vi "Production Mode Alt Gas.vi"() -> ()   [LabVIEW 2019]
uses:
  <vilib>/Instr/_visa.llb/VISA Configure Serial Port (Instr).vi
  <vilib>/regexp/Match Regular Expression.xnode
panel:
  in  "Gas Type":bool
  in  "Name":string
  in  "sMDT Code":string
  out "Previous\nTest Passed":bool
  out "Status":string
  in  "Start":bool
  out "Leak":string
  out "Pressure (mTorr)":dbl
  # "100% He"
  # "5% He"
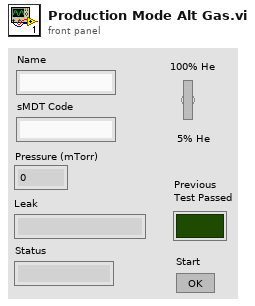
[diagram p1: front panel]
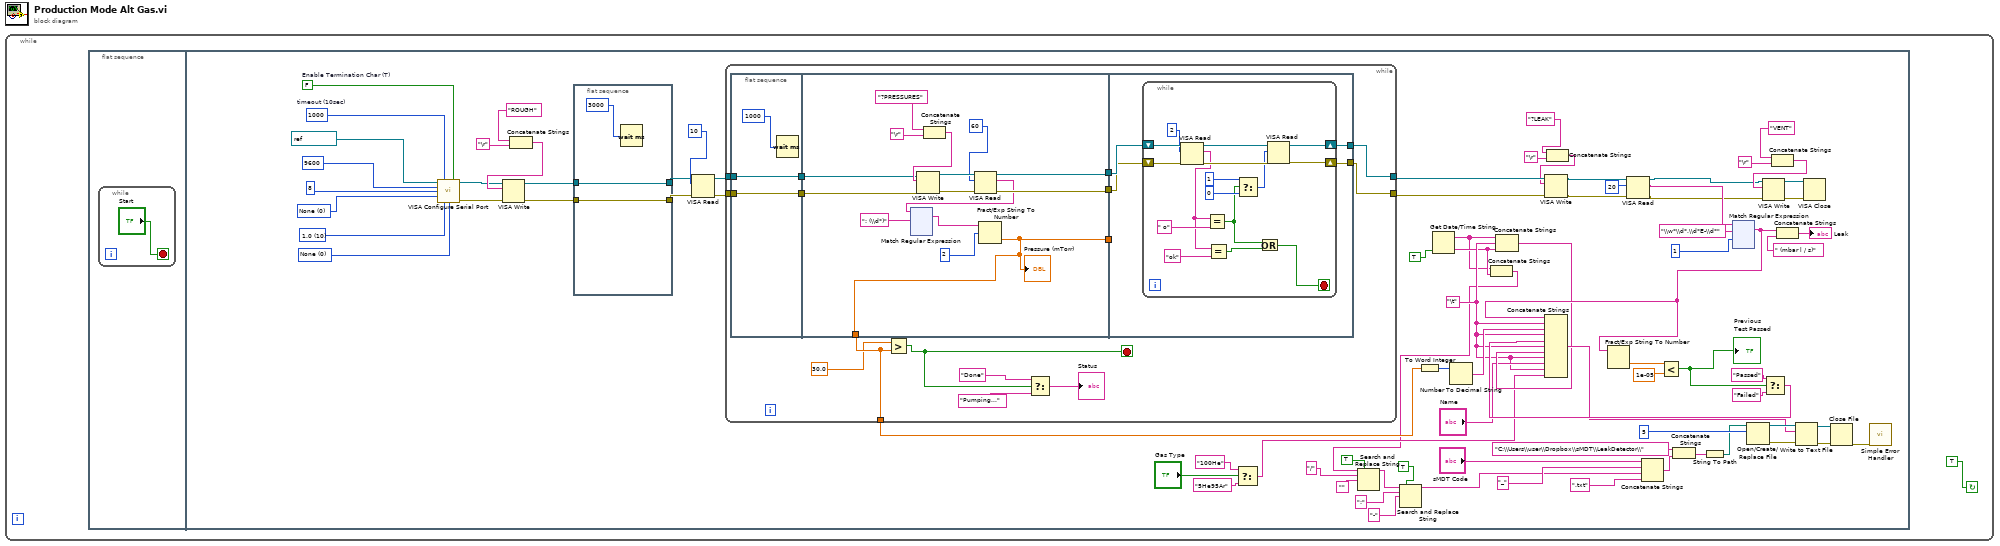
[diagram p0: block diagram]
diagram:
  n1 = while {
    stop <- TRUE continue-if-true
    n2 = flat-sequence {
      frame #0 {
        n3 = while {
          stop <- "Start" stop-if-true
        }
      }
      frame #1 {
        w16 = "\t"
        w79 = u16 0 items=["None"=0, "XON/XOFF"=1, "RTS/CTS"=2, "DTR/DSR"=4] ("flow control")
        w80 = u16 10 items=["1.0"=10, "1.5"=15, "2.0"=20] ("stop bits")
        w81 = u16 0 items=["None", "Odd", "Even", "Mark", "Space"] ("parity")
        w84 = FALSE  # Enable Termination Char (T)
        w85 = u32 1000  # timeout (10sec)
        n4 = call-poly "VISA Configure Serial Port"("VISA resource name"=refnum<visa-resource-name> "COM3", "timeout (10sec)"=w85, "Enable Termination\nChar (T)"=w84, "baud rate (9600)"=u32 9600 ("baud rate"), "data bits (8)"=u16 8 ("data bits"), "parity (0:none)"=w81, "stop bits (10: 1 bit)"=w80, "flow control (0:none)"=w79) -> ("VISA resource name out"=w18:refnum<visa-resource-name>, "error out"=w17:errorcluster)  [unwired: 6 in]
        n5 = Concatenate Strings("ROUGH", "\r") -> (w76:string)
        n6 = VISA Write(VISA resource name=w18, write buffer=w76, error in (no error)=w17) -> (VISA resource name out=w70:refnum<visa-resource-name>, error out=w69:errorcluster)  [unwired: 1 out]
        n7 = flat-sequence {
          tunnel: w70 -> [w367]
          tunnel: w69 -> [w368]
          tunnel: [w368] -> w66
          tunnel: [w367] -> w67
          frame #0 {
            n8 = Wait (ms)(milliseconds to wait=3000) -> ()  [unwired: 1 out]
          }
        }
        n9 = VISA Read(VISA resource name=w67, byte count=10, error in (no error)=w66) -> (VISA resource name out=w64:refnum<visa-resource-name>, error out=w65:errorcluster)  [unwired: 2 out]
        n10 = while {
          tunnel: w64 -> [w100]
          tunnel: w65 -> [w99]
          tunnel: [w88] -> w55
          tunnel: [w87] -> w54
          tunnel: [w92] -> w31
          stop <- w93 stop-if-true
          n11 = flat-sequence {
            tunnel: w100 -> [w103]
            tunnel: w99 -> [w102]
            tunnel: [w103] -> w98
            tunnel: [w102] -> w97
            tunnel: w98 -> [w112]
            tunnel: w97 -> [w111]
            tunnel: [w105] -> w92
            tunnel: [w109] -> w91
            tunnel: [w110] -> w90
            tunnel: [w105] -> w89
            tunnel: w91 -> [w235]
            tunnel: w90 -> [w236]
            tunnel: w89 -> [_]
            tunnel: [w234] -> w88
            tunnel: [w233] -> w87
            frame #0 {
              n12 = Wait (ms)(milliseconds to wait=1000) -> ()  [unwired: 1 out]
            }
            frame #1 {
              n13 = Concatenate Strings("?PRESSURES", "\r") -> (w113:string)
              n14 = VISA Write(VISA resource name=w112, write buffer=w113, error in (no error)=w111) -> (VISA resource name out=w118:refnum<visa-resource-name>, error out=w117:errorcluster)  [unwired: 1 out]
              n15 = VISA Read(VISA resource name=w118, byte count=60, error in (no error)=w117) -> (VISA resource name out=w110:refnum<visa-resource-name>, read buffer=w104:string, error out=w109:errorcluster)  [unwired: 1 out]
              n16 = xnode "Match Regular Expression"("input string"=w104, "regular expression"=": (\\d*)") -> ("whole match"=w108:string)  [unwired: 4 in, 4 out]
              n17 = Fract/Exp String To Number(string=w108, offset=2) -> (number=w105:dbl)  [unwired: 2 in, 1 out]
              "Pressure (mTorr)" <- w105
            }
            frame #2 {
              n18 = while {
                shift-right: [w246] -> w234
                shift-left: w236 -> [w252]
                shift-right: [w247] -> w233
                shift-left: w235 -> [w249]
                stop <- w237 stop-if-true
                n19 = VISA Read(VISA resource name=w252, byte count=2, error in (no error)=w249) -> (VISA resource name out=w250:refnum<visa-resource-name>, read buffer=w240:string, error out=w248:errorcluster)  [unwired: 1 out]
                n20 = Equal?(x=w240, y=" o") -> (x = y?=w238:bool)
                n21 = Equal?(x=w240, y="ok") -> (x = y?=w239:bool)
                n22 = Select(t=1, s=w238, f=0) -> (s? t:f=w243:i32)
                n23 = Or(x=w238, y=w239) -> (x .or. y?=w237:bool)
                n24 = VISA Read(VISA resource name=w250, byte count=w243, error in (no error)=w248) -> (VISA resource name out=w246:refnum<visa-resource-name>, error out=w247:errorcluster)  [unwired: 2 out]
              }
            }
          }
          n25 = Greater?(x=30.0 ("Pump Pressure"), y=w92) -> (0:w93:bool)
          n26 = Select(t="Done", s=w93, f="Pumping...") -> (s? t:f=→"Status":string)
        }
        n27 = Select(t="100He", s="Gas Type", f="5He95Ar") -> (s? t:f=w12:string)
        n28 = To Word Integer(number=w31) -> (16bit integer=w30:i16)
        n29 = Get Date/Time String(want seconds? (F)=TRUE) -> (date string=w9:string, time string=w10:string)  [unwired: 2 in]
        n30 = Number To Decimal String(number=w30) -> (decimal integer string=w27:string)  [unwired: 1 in]
        n31 = Concatenate Strings(w9, w10) -> (w8:string)
        n32 = Search and Replace String(replace all?=TRUE, input string=w8, search string="/", replace string="") -> (result string=w3:string)  [unwired: 4 in, 3 out]
        n33 = Search and Replace String(replace all?=TRUE, input string=w3, search string=":", replace string="-") -> (result string=w7:string)  [unwired: 4 in, 3 out]
        n34 = Concatenate Strings(w9, w16, w10) -> (w24:string)
        n35 = Concatenate Strings("?LEAK", "\r") -> (w51:string)
        n36 = VISA Write(VISA resource name=w55, write buffer=w51, error in (no error)=w54) -> (VISA resource name out=w50:refnum<visa-resource-name>, error out=w49:errorcluster)  [unwired: 1 out]
        n37 = VISA Read(VISA resource name=w50, byte count=20, error in (no error)=w49) -> (VISA resource name out=w57:refnum<visa-resource-name>, read buffer=w58:string, error out=w56:errorcluster)  [unwired: 1 out]
        n38 = Concatenate Strings("sMDT Code", "_", w7, ".txt") -> (w38:string)
        n39 = Concatenate Strings("C:\\Users\\user\\Dropbox\\sMDT\\LeakDetector\\", w38) -> (w22:string)
        n40 = String To Path(string=w22) -> (path=w40:path)
        n41 = xnode "Match Regular Expression"("input string"=w58, "regular expression"="\\w*\\d*.\\d*E-\\d*", "offset (0)"=1) -> ("whole match"=w35:string)  [unwired: 3 in, 4 out]
        n42 = Fract/Exp String To Number(string=w35) -> (number=w47:dbl)  [unwired: 3 in, 1 out]
        n43 = Less?(x=w47, y=1e-05) -> (x < y?=w33:bool)
        "Previous\nTest Passed" <- w33
        n44 = Open/Create/Replace File(file path (use dialog)=w40, operation (0:open)=5) -> (refnum out=w45:refnum<file>, error out=w43:errorcluster)  [unwired: 4 in, 1 out]
        n45 = Select(t="Passed", s=w33, f="Failed") -> (s? t:f=w26:string)
        n46 = Concatenate Strings(w35, w16, w27, w16, w26, w16, w24, w16, "Name", w16, w12) -> (w25:string)
        n47 = Concatenate Strings("VENT", "\r") -> (w73:string)
        n48 = VISA Write(VISA resource name=w57, write buffer=w73, error in (no error)=w56) -> (VISA resource name out=w72:refnum<visa-resource-name>, error out=w71:errorcluster)  [unwired: 1 out]
        n49 = Concatenate Strings(w35, " (mbar l / s)") -> (→"Leak":string)
        n50 = Write to Text File(file (use dialog)=w45, text=w25, error in=w43) -> (refnum out=w44:refnum<file>, error out=w42:errorcluster)  [unwired: 1 in, 1 out]
        n51 = VISA Close(VISA resource name=w72, error in (no error)=w71) -> ()  [unwired: 1 out]
        n52 = Close File(refnum=w44, error in=w42) -> (error out=w41:errorcluster)  [unwired: 1 out]
        n53 = call <vilib>:"Simple Error Handler.vi"("error in (no error)"=w41) -> ()  [unwired: 4 in, 5 out]
      }
    }
  }
